vi "test.vi"() -> ()   [LabVIEW 2021]
uses:
  Measurement Configuration.ctl
  <vilib>/PDM Acquisition Toolkit/host/Classes/Tasks/PCM Input/Controls/DVR PCM Input Task.ctl
  <vilib>/PDM Acquisition Toolkit/host/Classes/Tasks/PCM Input/PCM Input Task.lvclass
  <vilib>/PDM Acquisition Toolkit/host/API/Public/Start/Start PCM Input Task.vi
  <vilib>/PDM Acquisition Toolkit/host/API/Public/Read/Read PCM Input Waveform.vi
  <vilib>/PDM Acquisition Toolkit/host/API/Public/Stop/Stop PCM Input Task.vi
  <vilib>/PDM Acquisition Toolkit/host/API/Public/Clear/Clear PCM Input Task.vi
  <vilib>/PDM Acquisition Toolkit/host/API/PDM Acquisition Toolkit.lvlib
panel:
  out "Waveform Graph 2":dbl[](graph)
  out "size time":i32
  out "size spectrum":i32
  out "TimeDomain":dbl[](array[numeric])
  out "Spectrum":dbl[](array[numeric])
  in  "WeightingFilter":string
  out "size(s)":i32
  in  "MeasurementConfiguration":T1={"BandStart"=20.0, "BandStop"=20000.0, "Amplitude"=1.0, "Frequency"=1000.0, "FullScaleRange"=2.825, "DataLine"=0, "SampleRate"=12288000, "MeasurementDuration"=19200.0, "Channel"=0, "FrameSyncEdgeForChannel_0"=0, "ChannelCountPerFrame"=2, "ChannelLength"=32, "BitDepth"=24, "Channel_0_offset"=1, "Endianness"=0, "DataJustification"=0, "FrameSyncPulseWidth"=32, "BitClockEdgeSync"=1, "ClockRate"=0, "FrameLength"=0, "NumberOfWords"=0, "Sensitivity"=0.0} {"MeasurementDuration" format="%.1f"}
  in  "ProtocolCaptureResourceName":string
  out "Y":dbl[](array[numeric])
  out "dt":dbl
  out "Waveform Graph":waveform(dbl)(graph)
  out "error out":errorcluster
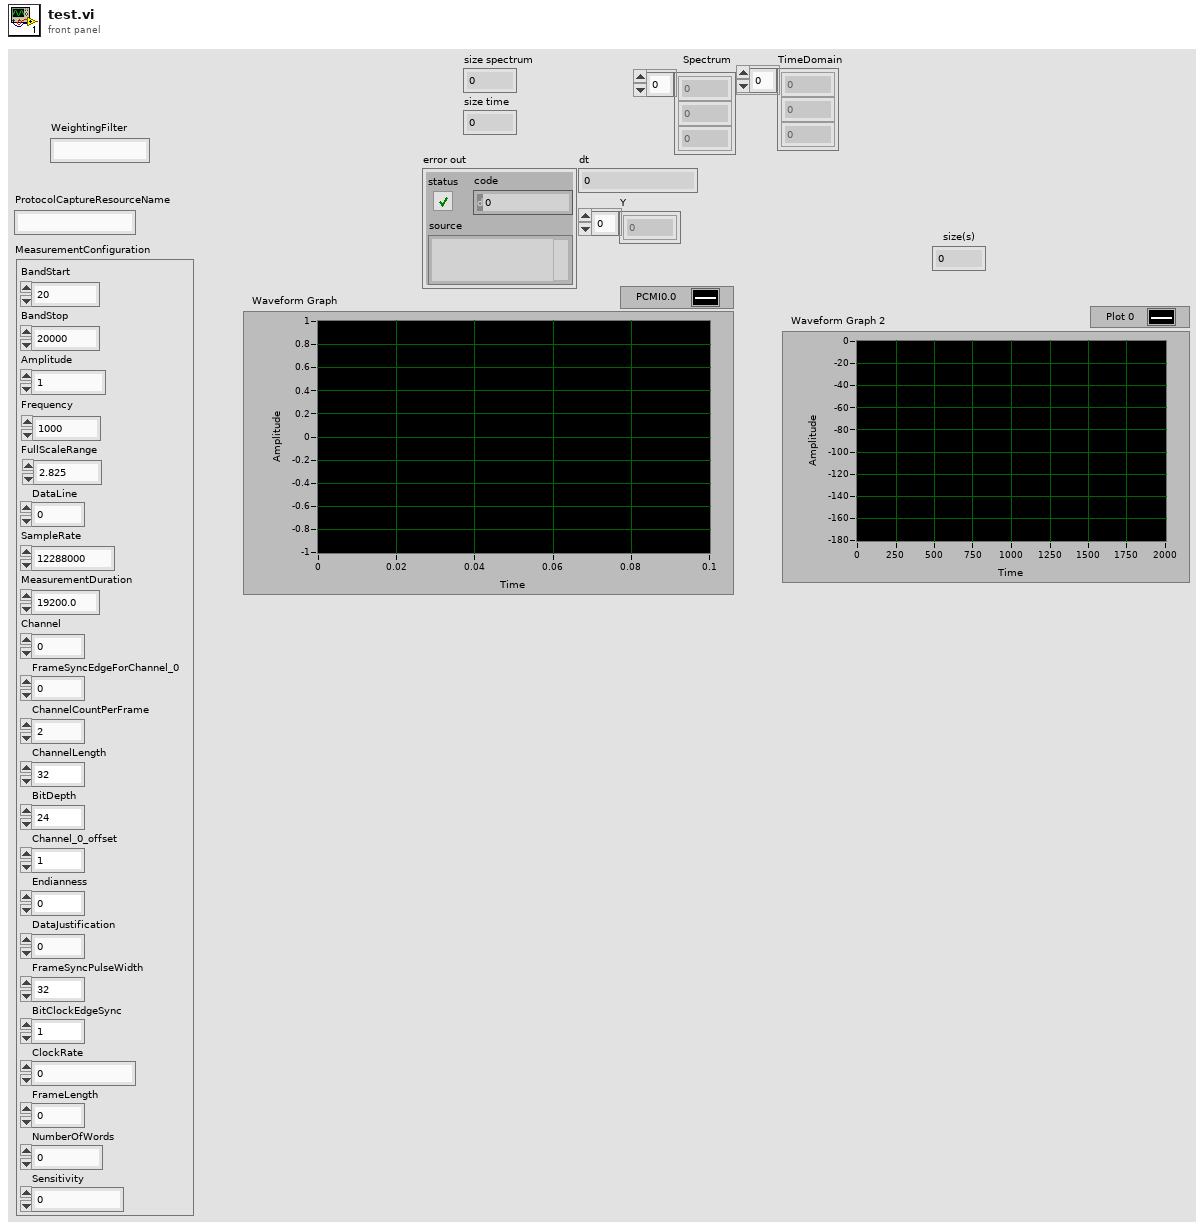
[diagram p1: front panel]
types:
  T1 = typedef "Measurement Configuration.ctl" = cluster{"BandStart":dbl, "BandStop":dbl, "Amplitude":dbl, "Frequency":dbl, "FullScaleRange":dbl, "DataLine":u32, "SampleRate":u32, "MeasurementDuration":dbl, "Channel":u32, "FrameSyncEdgeForChannel_0":u32, "ChannelCountPerFrame":u32, "ChannelLength":u32, "BitDepth":u32, "Channel_0_offset":u32, "Endianness":u32, "DataJustification":u32, "FrameSyncPulseWidth":u32, "BitClockEdgeSync":u32, "ClockRate":u32, "FrameLength":u32, "NumberOfWords":u32, "Sensitivity":dbl}
  T2 = typedef "PDM Acquisition Class Library.lvlib/PCM Input Task.lvclass/DVR PCM Input Task.ctl" = refnum<data-value>
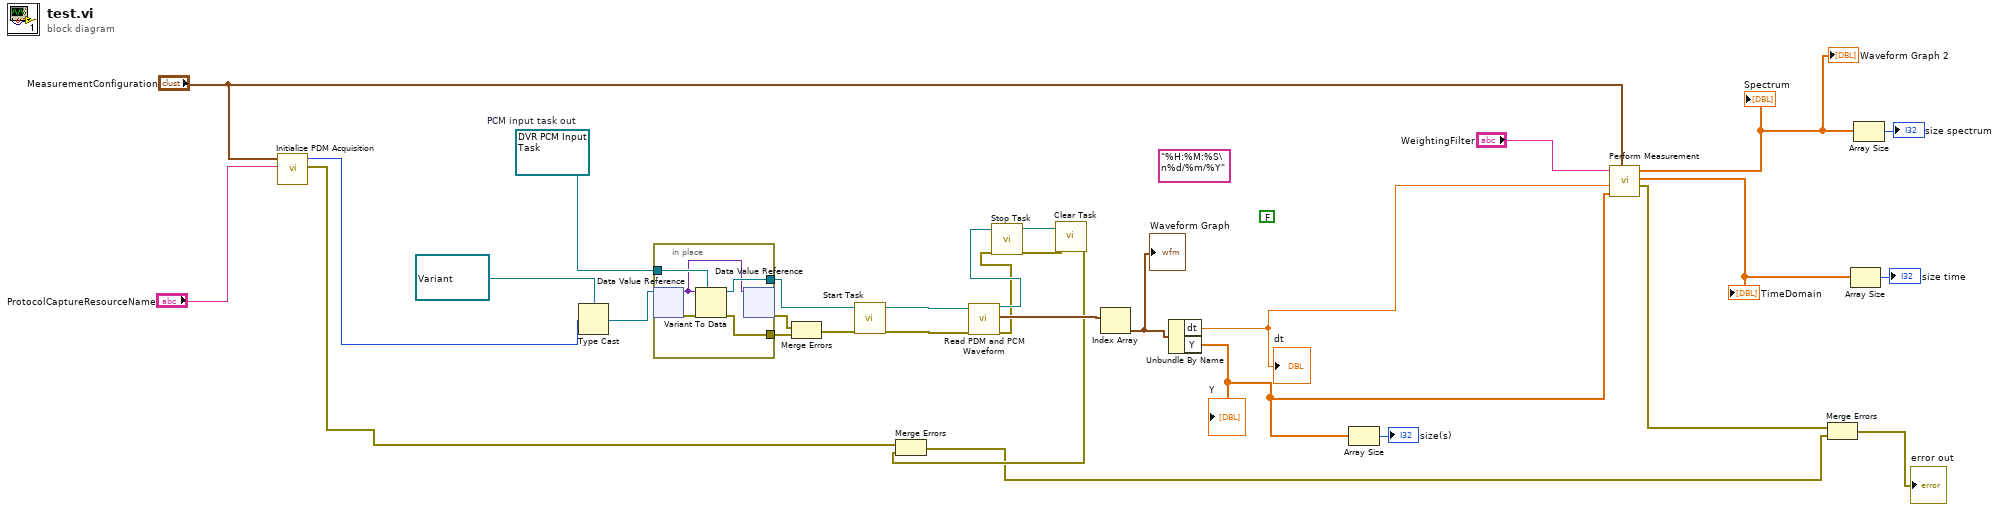
[diagram p0: block diagram]
diagram:
  (unwired) "%H:%M:%S\n%d/%m/%Y" ("time format string (%c)")
  (unwired) FALSE ("UTC format")
  w26 = T2 refnum  # PCM input task out
  n1 = call "Initialize PDM Acquisition.vi"("ProtocolCaptureResourceName"="ProtocolCaptureResourceName", "MeasurementConfiguration"="MeasurementConfiguration") -> ("error out"=w18:errorcluster, "ObjRefOut"=w19:u32)  [unwired: 7 in]
  n2 = Type Cast(type=refnum<data-value> refnum ("data value reference"), x=w19) -> (*(type *) &x=w24:refnum<data-value>)
  n3 = in-place {
    in-place-border: [w36] -> w25
    in-place-border: [w34] -> w29
    in-place-border: w26 -> [w33]
    n4 = in-place-dvr #1(w24) -> (w32:variant, w35:errorcluster)
    n5 = Variant To Data(error in=w35, type=w33, Variant=w32) -> (data=w36:T2, error out=w34:errorcluster)
    n6 = in-place-dvr #1(w32) -> (w30:errorcluster)  [unwired: 1 out]
  }
  n7 = Merge Errors(w30, w29) -> (w28:errorcluster)
  n8 = call-poly <vilib>:"Start Task.vi"("error in"=w28, "PCM input task in"=w25) -> ("error out"=w31:errorcluster, "PCM input task out"=w27:T2)  [unwired: 8 in]
  n9 = call-poly <vilib>:"Read PDM and PCM Waveform.vi"("error in"=w31, "PCM input task In"=w27) -> ("error out"=w6:errorcluster, "PCM waveforms"=w22:waveform(dbl)[], "PCM input task out"=w8:T2)  [unwired: 4 in, 3 out]
  n10 = call-poly <vilib>:"Stop Task.vi"("error in"=w6, "PCM input task In"=w8) -> ("error out"=w5:errorcluster, "PCM input task out"=w7:T2)  [unwired: 8 in]
  n11 = call-poly <vilib>:"Clear Task.vi"("error in"=w5, "PCM input task in"=w7) -> ("error out"=w4:errorcluster)  [unwired: 9 in]
  n12 = Merge Errors(w18, w4) -> (w3:errorcluster)
  n13 = Index Array(array=w22) -> (element=w21:waveform(dbl))  [unwired: 1 in]
  "Waveform Graph" <- w21
  n14 = Unbundle By Name(w21) -> ("dt"=w15:dbl, "Y"=w14:dbl[])
  "dt" <- w15
  "Y" <- w14
  n15 = Array Size(array=w14) -> (size(s)=→"size(s)":i32)
  n16 = call "Perform Measurement.vi"("MeasurementConfiguration"="MeasurementConfiguration", "Y"=w14, "dt"=w15, "WeightingFilter"="WeightingFilter") -> ("error out"=w2:errorcluster, "TimeDomain"=w12:dbl[], "Spectrum"=w9:dbl[])  [unwired: 4 in, 1 out]
  "Spectrum" <- w9
  "TimeDomain" <- w12
  "Waveform Graph 2" <- w9
  n17 = Merge Errors(w2, w3) -> (→"error out":errorcluster)
  n18 = Array Size(array=w12) -> (size(s)=→"size time":i32)
  n19 = Array Size(array=w9) -> (size(s)=→"size spectrum":i32)
